vi "Vertical speed (SubVI).vi"(11 "Array of Joint Positions in":dbl[][](array[numeric])=[[-0.12146424502134323, 0.001454623183235526, 1.9073543548583984], [-0.11488837748765945, 0.05537768453359604, 1.9802660942077637], [-0.11157815903425217, 0.43785253167152405, 2.0466103553771973], [-0.1483002007007599, 0.6516268253326416, 2.0609679222106934], [-0.30285415053367615, 0.2956160008907318, 2.029113531112671], [-0.38003623485565186, 0.031045880168676376, 1.9445093870162964], [-0.35092946887016296, -0.1451244205236435, 1.7685273885726929], [-0.3320053219795227, -0.2223913073539734, 1.670140027999878], [0.04304381087422371, 0.29154613614082336, 1.9958680868148804], [0.13985766470432281, 0.025840533897280693, 1.922817349433899], [0.12575246393680573, -0.14097267389297485, 1.7425767183303833], [0.10289721190929413, -0.2135094851255417, 1.649812936782837], [-0.1967616081237793, -0.07389465719461441, 1.8869941234588623], [-0.2406357079744339, -0.5076637864112854, 1.838017225265503], [-0.23708361387252808, -0.8213208913803101, 1.8209781646728516], [-0.24613811075687408, -0.8672351241111755, 1.7265561819076538], [-0.04989041015505791, -0.0703207477927208, 1.876594066619873], [-0.015257264487445354, -0.5077733993530273, 1.839611291885376], [-0.002423219382762909, -0.818880021572113, 1.8193140029907227], [-0.007616172078996897, -0.8644676804542542, 1.7244435548782349]]) -> (2 "x .and. y?":bool, 3 "Vertical Speed":dbl)   [LabVIEW 2014]
uses:
  Kinect Global.vi
  <vilib>/Analysis/NI_AALPro.lvlib
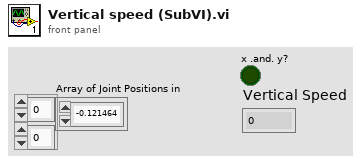
[diagram p1: front panel]
types:
  T1 = enum16{"hip centre", "spine", "shoulder centre", "head", "shoulder left", "elbow left", "wrist left", "hand left", "shoulder right", "elbow right", "wrist right", "hand right", "hip left", "knee left", "ankle left", "foot left", "hip right", "knee right", "ankle right", "foot right"}
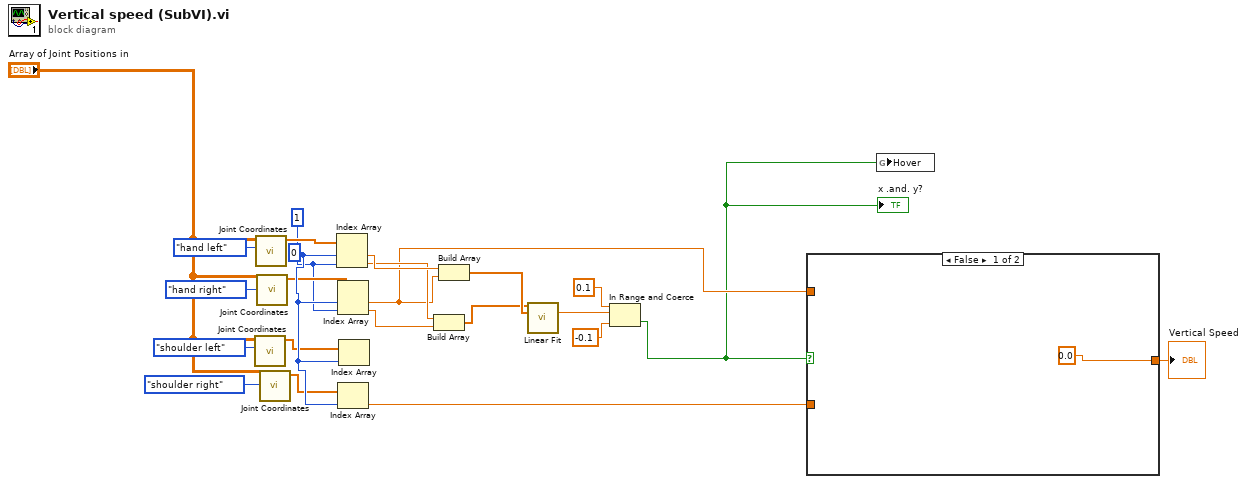
[diagram p0: block diagram]
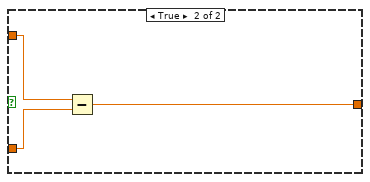
[diagram p2: hidden frame]
diagram:
  w13 = 1 ("index")
  w22 = 0 ("index")
  n1 = call <vilib>:"Joint Coordinates.vi"("Joint 1"=T1."shoulder left", "Array of Joint Positions"="Array of Joint Positions in") -> ("Joint Coordinates"=w20:dbl[])  [unwired: 8 in, 1 out]
  n2 = call <vilib>:"Joint Coordinates.vi"("Joint 1"=T1."hand left", "Array of Joint Positions"="Array of Joint Positions in") -> ("Joint Coordinates"=w18:dbl[])  [unwired: 8 in, 1 out]
  n3 = call <vilib>:"Joint Coordinates.vi"("Joint 1"=T1."hand right" ("Joint 2"), "Array of Joint Positions"="Array of Joint Positions in") -> ("Joint Coordinates"=w19:dbl[])  [unwired: 8 in, 1 out]
  n4 = call <vilib>:"Joint Coordinates.vi"("Joint 1"=T1."shoulder right" ("Joint 2"), "Array of Joint Positions"="Array of Joint Positions in") -> ("Joint Coordinates"=w21:dbl[])  [unwired: 8 in, 1 out]
  n5 = Index Array(array=w18, index #1=w22, index #2=w13) -> (element #1=w12:dbl, element #2=w11:dbl)
  n6 = Index Array(array=w19, index #1=w22, index #2=w13) -> (element #1=w4:dbl, element #2=w10:dbl)
  n7 = Index Array(array=w21, index=w22) -> (element=w3:dbl)
  n8 = Index Array(array=w20, index=w22) -> ()  [unwired: 1 out]
  n9 = Build Array(w11, w10) -> (w8:dbl[])
  n10 = Build Array(w12, w4) -> (w9:dbl[])
  n11 = call <vilib>:"Linear Fit.vi"("Y"=w8, "X"=w9) -> ("slope"=w7:dbl)  [unwired: 9 in, 4 out]
  n12 = In Range and Coerce(upper limit=0.1, x=w7, lower limit=-0.1) -> (In Range?=w1:bool)  [unwired: 1 out]
  "x .and. y?" <- w1
  n13 = case shown="False" w1 {
    tunnel: w4 -> [_ w27]
    tunnel: w3 -> [_ w26]
    tunnel: [0.0 w25] -> w2
    frame False {
    }
    frame True {
      n14 = Subtract(x=w27, y=w26) -> (x-y=w25:dbl)
    }
  }
  "Vertical Speed" <- w2
  n15 = global write "Kinect Global.vi" "Hover"(w1) -> ()
